vi "CmdCode2Elements.vi"(2 "error in (no error)":errorcluster, 3 "CommandCode":string) -> (0 "error out":errorcluster, 1 "Elements":T1)   [LabVIEW 2010]
uses:
  <vilib>/regexp/Match Regular Expression.xnode
panel:
  out "whole match":string
  in  "regular expression":string="68[0-9ABCDEF]{12}68[0-9ABCDEF]{8,}16"
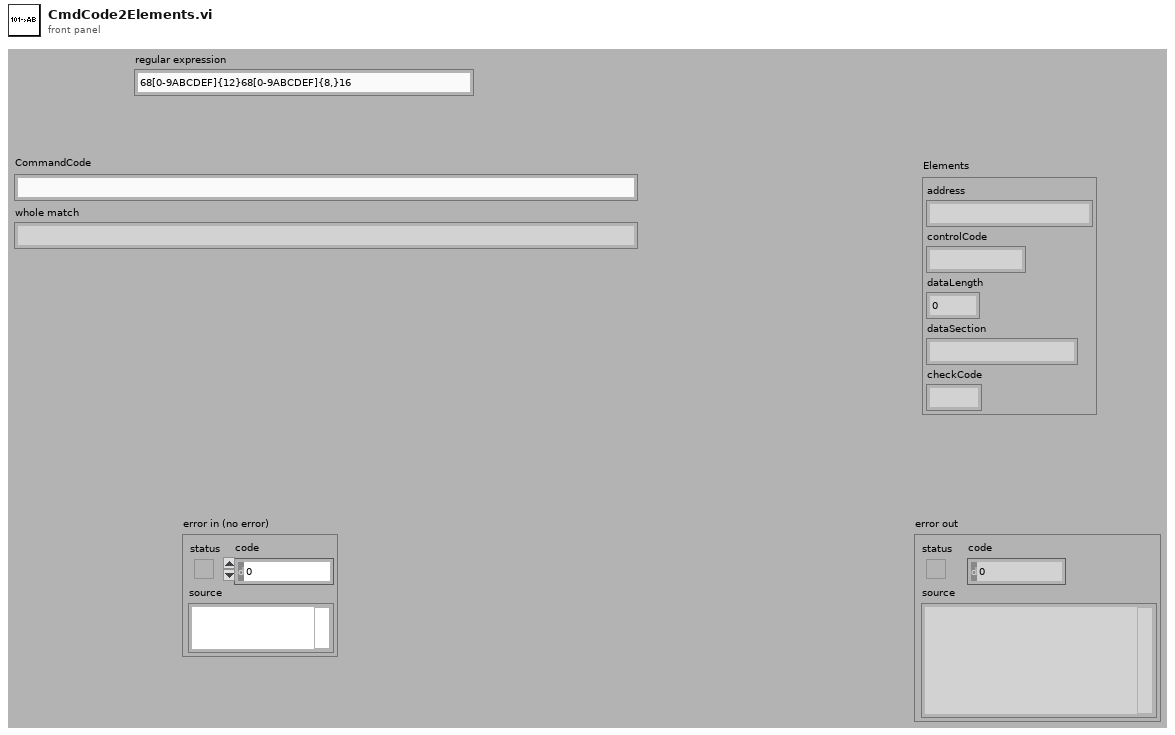
[diagram p1: front panel]
types:
  T1 = cluster{"address":string, "controlCode":string, "dataLength":dbl, "dataSection":string, "checkCode":string}
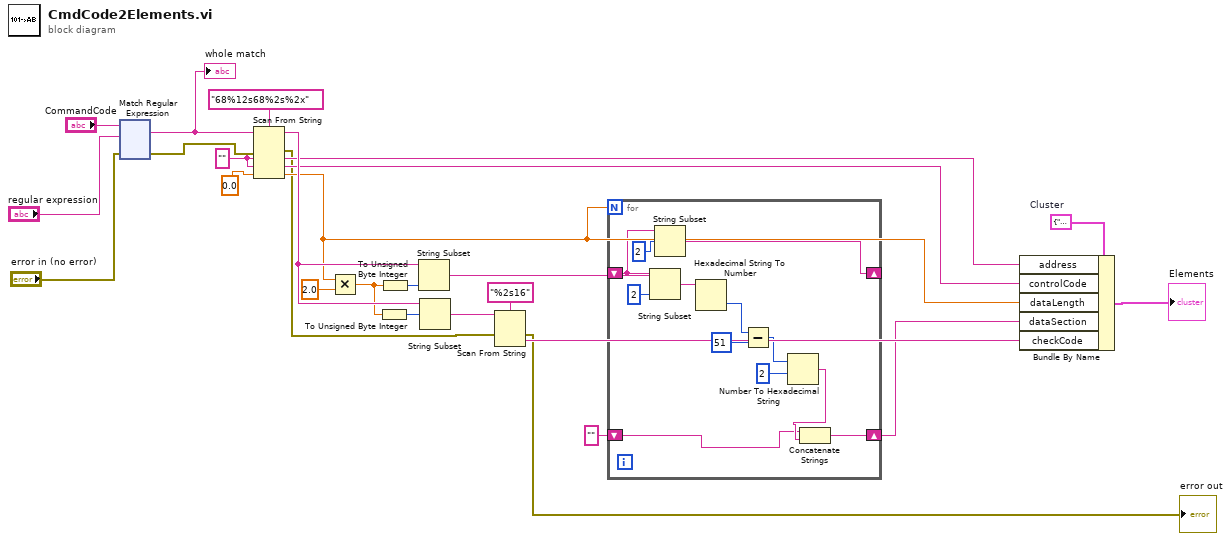
[diagram p0: block diagram]
diagram:
  w12 = T1 {"address"="100000000000", "controlCode"="15", "dataLength"=12.0, "dataSection"="343333333333", "checkCode"="47"}  # Cluster
  w23 = "" ("default value 1")
  n1 = xnode "Match Regular Expression"("input string"="CommandCode", "regular expression"="regular expression", "error in"="error in (no error)") -> ("whole match"=w24:string, "error out"=w3:errorcluster)  [unwired: 3 in, 3 out]
  "whole match" <- w24
  n2 = Scan From String(format string="68%12s68%2s%2x", input string=w24, error in=w3, default 1=w23, default 2=w23, default 3=0.0) -> (remaining string=w20:string, error out=w2:errorcluster, output 1=w15:string, output 2=w14:string, output 3=w8:dbl)  [unwired: 1 in, 1 out]
  n3 = Multiply(x=w8, y=2.0) -> (x*y=w10:dbl)
  n4 = To Unsigned Byte Integer(number=w10) -> (unsigned 8bit integer=w18:u8)
  n5 = To Unsigned Byte Integer(number=w10) -> (unsigned 8bit integer=w19:u8)
  n6 = String Subset(string=w20, length (rest)=w19) -> (substring=w7:string)  [unwired: 1 in]
  n7 = String Subset(string=w20, offset (0)=w18) -> (substring=w17:string)  [unwired: 1 in]
  n8 = Scan From String(format string="%2s16", input string=w17, error in=w2) -> (error out=→"error out":errorcluster, output 1=w13:string)  [unwired: 2 in, 2 out]
  n9 = for {
    N: w8 -> [_]
    shift-right: [w32] -> _
    shift-left: w7 -> [w33]
    shift-right: [w31] -> w6
    shift-left: "" -> [w27]
    n10 = String Subset(string=w33, length (rest)=2 ("长度（剩余）")) -> (substring=w38:string)  [unwired: 1 in]
    n11 = String Subset(string=w33, offset (0)=2 ("长度（剩余）")) -> (substring=w32:string)  [unwired: 1 in]
    n12 = Hexadecimal String To Number(string=w38) -> (number=w37:u32)  [unwired: 2 in, 1 out]
    n13 = Subtract(x=w37, y=u32 51) -> (x-y=w35:u32)
    n14 = Number To Hexadecimal String(1:i16 2 ("宽度(-)"), 2:w35) -> (0:w28:string)
    n15 = Concatenate Strings(w27, w28) -> (w31:string)
  }
  n16 = Bundle By Name(cluster=w12, "address"=w15, "controlCode"=w14, "dataLength"=w8, "dataSection"=w6, "checkCode"=w13) -> (→"Elements":T1)
